vi "VXM_MotorPositionF.vi"() -> (3 "Position":i32[](array[numeric]))   [LabVIEW 2020]
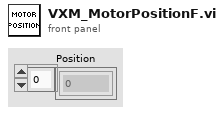
[diagram p1: front panel]
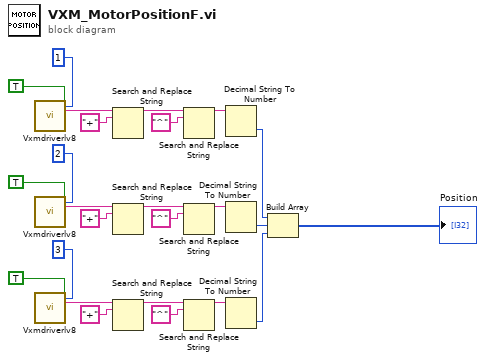
[diagram p0: block diagram]
diagram:
  n1 = call "Vxmdriverlv8.Vi"("Get\nMotor\nPosition"=TRUE ("Get\nMotor\nPosition"), "Motor\nNumber"=1 ("Motor\nNumber")) -> ("Motor Position"=w14:string)  [unwired: 20 in, 5 out]
  n2 = call "Vxmdriverlv8.Vi"("Get\nMotor\nPosition"=TRUE ("Get\nMotor\nPosition"), "Motor\nNumber"=2 ("Motor\nNumber")) -> ("Motor Position"=w2:string)  [unwired: 20 in, 5 out]
  n3 = call "Vxmdriverlv8.Vi"("Get\nMotor\nPosition"=TRUE ("Get\nMotor\nPosition"), "Motor\nNumber"=3 ("Motor\nNumber")) -> ("Motor Position"=w5:string)  [unwired: 20 in, 5 out]
  n4 = Search and Replace String(input string=w14, search string="+") -> (result string=w16:string)  [unwired: 6 in, 3 out]
  n5 = Search and Replace String(input string=w2, search string="+") -> (result string=w11:string)  [unwired: 6 in, 3 out]
  n6 = Search and Replace String(input string=w5, search string="+") -> (result string=w8:string)  [unwired: 6 in, 3 out]
  n7 = Search and Replace String(input string=w16, search string="^") -> (result string=w12:string)  [unwired: 6 in, 3 out]
  n8 = Search and Replace String(input string=w11, search string="^") -> (result string=w3:string)  [unwired: 6 in, 3 out]
  n9 = Search and Replace String(input string=w8, search string="^") -> (result string=w4:string)  [unwired: 6 in, 3 out]
  n10 = Decimal String To Number(string=w12) -> (number=w1:i32)  [unwired: 2 in, 1 out]
  n11 = Decimal String To Number(string=w3) -> (number=w19:i32)  [unwired: 2 in, 1 out]
  n12 = Decimal String To Number(string=w4) -> (number=w18:i32)  [unwired: 2 in, 1 out]
  n13 = Build Array(w1, w19, w18) -> (→"Position":i32[])
